vi "CommandLine.vi"(11 "Table limits":T1) -> (3 "Command line":string)   [LabVIEW 2023]
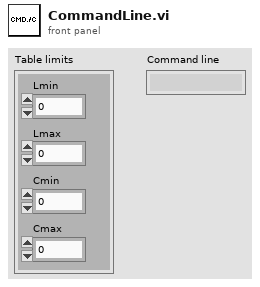
[diagram p1: front panel]
types:
  T1 = cluster{"Lmin":i32, "Lmax":i32, "Cmin":i32, "Cmax":i32}
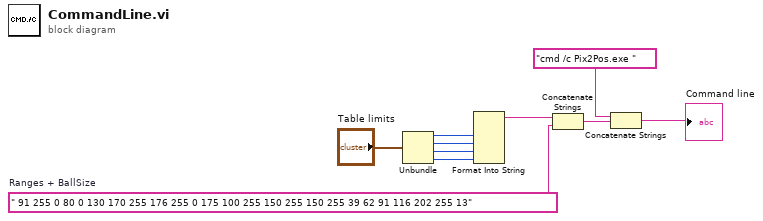
[diagram p0: block diagram]
diagram:
  w4 = " 91 255 0 80 0 130 170 255 176 255 0 175 100 255 150 255 150 255 39 62 91 116 202 255 13"  # Ranges + BallSize
  n1 = Unbundle("Table limits") -> ("Lmin"=w9:i32, "Lmax"=w8:i32, "Cmin"=w7:i32, "Cmax"=w6:i32)
  n2 = Format Into String(w9, w8, w7, w6) -> (resulting string=w5:string)  [unwired: 3 in, 1 out]
  n3 = Concatenate Strings(w5, w4) -> (w2:string)
  n4 = Concatenate Strings("cmd /c Pix2Pos.exe ", w2) -> (→"Command line":string)
